vi "Differential_delay_line_conf_Mezzaninev56.vi"(0 "connection ID":refnum<k5>, 5 "channel":i32, 7 "Delay value":u16, 9 "Id in":i32, 11 "error in (no error)":errorcluster) -> (4 "connection ID out":refnum<k5>, 6 "data read value 18":u32, 8 "data out serial 18":string, 10 "Data to send hex 18":string, 12 "Delay value out":u16(ring) items=["0", "0.25ns", "0.5ns", "0.75ns", "1ns", "1.25ns", "1.5ns", "1.75ns", "2ns", "2.25ns", "2.5ns", "2.75ns", "3ns", "3.25ns", "3.5ns", "3.75ns", "4ns", "4.25ns", "4.5ns", "4.75ns", "5ns", "5.25ns", "5.5ns", "5.75ns", "2ns_b", "2.25ns_b", "2.5ns_b", "2.75ns_b", "3ns_b", "3.25ns_b", "3.5ns_b", "3.75ns_b", ""], 13 "Value hex":u32, 14 "Id out":i32, 15 "error out 2":errorcluster)   [LabVIEW 2012]
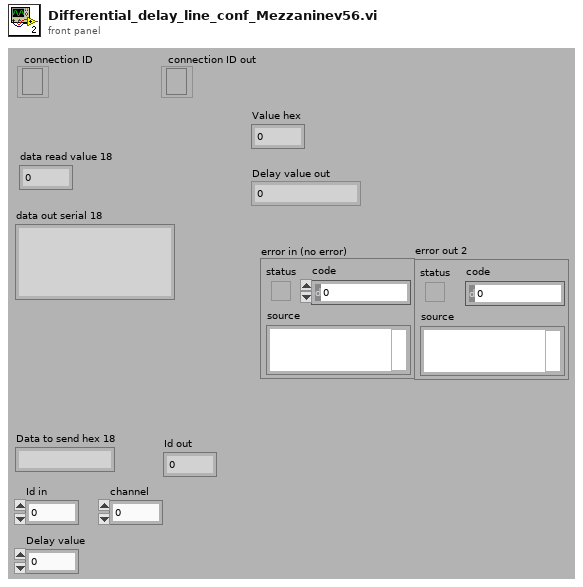
[diagram p1: front panel]
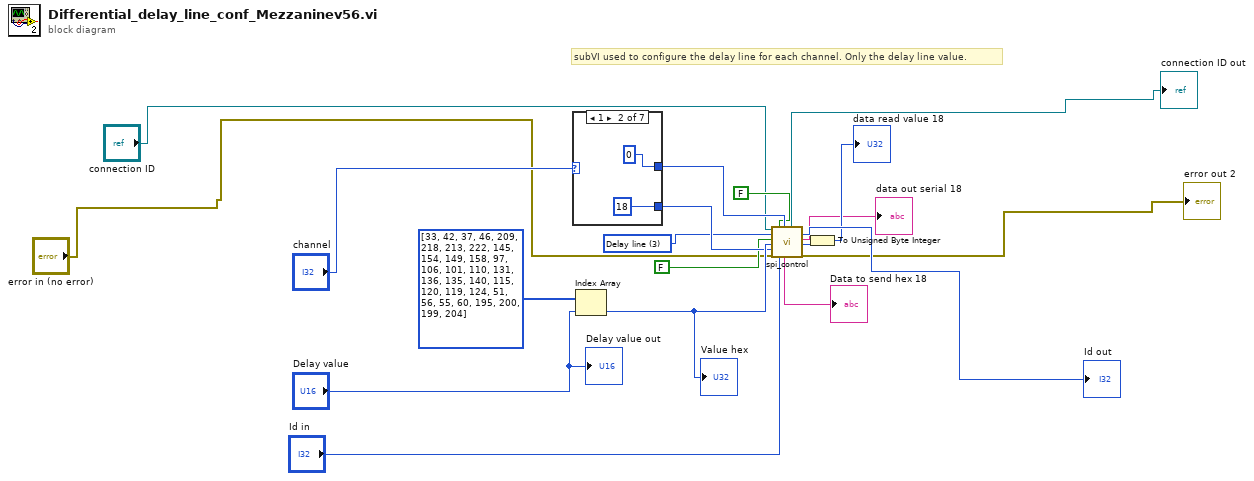
[diagram p0: block diagram]
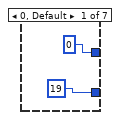
[diagram p2: hidden frame]
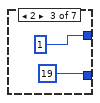
[diagram p3: hidden frame]
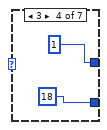
[diagram p4: hidden frame]
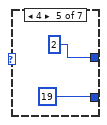
[diagram p5: hidden frame]
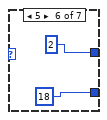
[diagram p6: hidden frame]
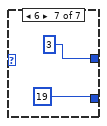
[diagram p7: hidden frame]
diagram:
  w7 = u16 3 items=["Attenuation", "Clipping", "Enable channel", "Delay line", "ASIC"] ("Device")
  # "subVI used to configure the delay line for each channel. Only the delay line value."
  n1 = case shown="1" "channel" {
    tunnel: [19 ("Register or channel") 18 ("Register or channel") 19 ("Register or channel") 18 ("Register or channel") 19 ("Register or channel") 18 ("Register or channel") 19 ("Register or channel")] -> w8
    tunnel: [0 ("Register or channel") 0 ("Register or channel") 1 ("Register or channel") 1 ("Register or channel") 2 ("Register or channel") 2 ("Register or channel") 3 ("Register or channel")] -> w11
    frame 0, Default {
    }
    frame 1 {
    }
    frame 2 {
    }
    frame 3 {
    }
    frame 4 {
    }
    frame 5 {
    }
    frame 6 {
    }
  }
  n2 = Index Array(array=u32[] [33, 42, 37, 46, 209, 218, 213, 222, 145, 154, 149, 158, 97, 106, 101, 110, 131, 136, 135, 140, 115, 120, 119, 124, 51, 56, 55, 60, 195, 200, 199, 204], index="Delay value") -> (element=w17:u32)
  "Value hex" <- w17
  n3 = call "spi_control.vi"("connection ID"="connection ID", "Device"=w7, "Read/#write"=FALSE, "Data"=w17, "Register or channel"=w8, "error out 3"="error in (no error)", "Read physical"=FALSE, "Id in"="Id in", "chip delay"=w11) -> ("Data to send hex"=→"Data to send hex 18":string, "connection ID out"=→"connection ID out":refnum<k5>, "Id out"=→"Id out":i32, "data out serial"=→"data out serial 18":string, "data read value"=w12:u32, "error out 2"=→"error out 2":errorcluster)  [unwired: 3 in, 2 out]
  n4 = To Unsigned Byte Integer(number=w12) -> (unsigned 8bit integer=→"data read value 18":u8)
  "Delay value out" <- "Delay value"
